vi "MovCor-Modify simulated DAQ sequence.vi"(10 "Number of POI":i32, 11 "Simulated control timings sequence in":waveform(dbl)) -> (3 "Simulated control timings sequence":waveform(dbl))   [LabVIEW 2020]
uses:
  Global Variables/General Globals.vi
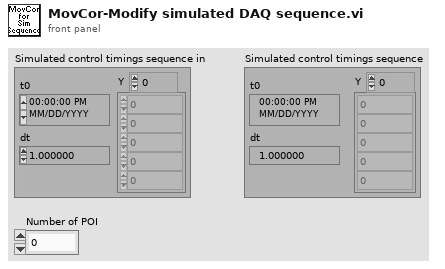
[diagram p1: front panel]
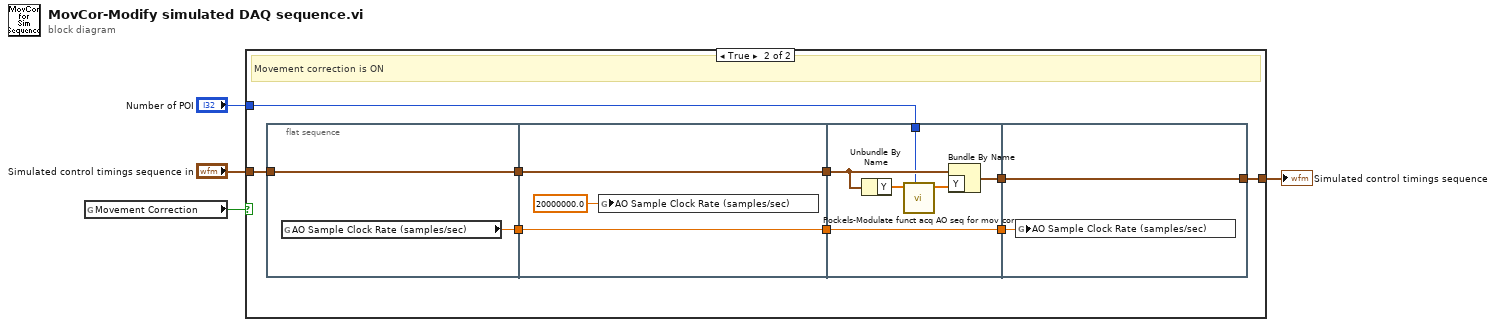
[diagram p0: block diagram]
diagram:
  n1 = global read "General Globals.vi" "Movement Correction"() -> (w2:bool)
  n2 = case shown="True" w2 {
    tunnel: "Simulated control timings sequence in" -> [w5 w14]
    tunnel: [w5 w13] -> w4
    tunnel: "Number of POI" -> [_ w6]
    frame False {
      # "Movement correction is OFF"
    }
    frame True {
      # "Movement correction is ON"
      n3 = flat-sequence {
        tunnel: w14 -> [w16]
        tunnel: [w16] -> w11
        tunnel: [w15] -> w9
        tunnel: w11 -> [w19]
        tunnel: [w19] -> w10
        tunnel: w9 -> [w18]
        tunnel: [w18] -> w8
        tunnel: [w22] -> w12
        tunnel: w10 -> [w25]
        tunnel: w8 -> [w21]
        tunnel: [w21] -> w7
        tunnel: w6 -> [w20]
        tunnel: [w27] -> w13
        tunnel: w12 -> [w27]
        tunnel: w7 -> [w26]
        frame #0 {
          n4 = global read "General Globals.vi" "AO Sample Clock Rate (samples/sec)"() -> (w15:dbl)
        }
        frame #1 {
          n5 = global write "General Globals.vi" "AO Sample Clock Rate (samples/sec)"(20000000.0 ("AO Sample Clock Rate (samples/sec)")) -> ()
        }
        frame #2 {
          n6 = Unbundle By Name(w25) -> ("Y"=w24:dbl[])
          n7 = call "Pockels-Modulate funct acq AO seq for mov cor.vi"("Number of POI"=w20, "Pockels modulation sequence in"=w24) -> ("Pockels modulation sequence out"=w23:dbl[])  [unwired: 8 in, 1 out]
          n8 = Bundle By Name(cluster=w25, "Y"=w23) -> (w22:waveform(dbl))
        }
        frame #3 {
          n9 = global write "General Globals.vi" "AO Sample Clock Rate (samples/sec)"(w26) -> ()
        }
      }
    }
  }
  "Simulated control timings sequence" <- w4
